vi "Msg Inspect.vi"(9 "From Msg Event":bool, 10 "Msg in":refnum<class "Msg.lvclass">, 11 "Base Actor in":refnum<class "Base Actor.lvclass">) -> (2 "Msg out":refnum<class "Msg.lvclass">, 3 "Base Actor out":refnum<class "Base Actor.lvclass">)   [LabVIEW 2020, in "jettl.lvlib" / "Actor.lvlib" / "Base Actor.lvclass"]
uses:
  Base Actor.lvclass
  Msg/Msg.lvclass
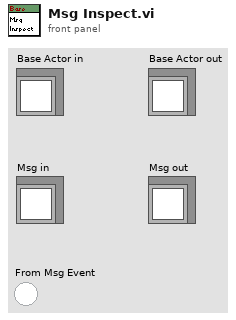
[diagram p1: front panel]
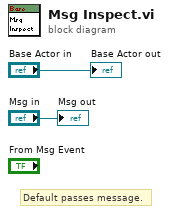
[diagram p0: block diagram]
diagram:
  # "Default passes message."
  "Base Actor out" <- "Base Actor in"
  "Msg out" <- "Msg in"
